vi "Write Qual and SData Masks.vi"(0 "private data":T1={"GTX2_CHANNEL register map"=refnum, "instruction target"=refnum, "channel measure state"=enum."Uninitialized", "in DFE mode?"=FALSE, "prescale"=0, "rx internal data width"=enum."32 Bit", "active point"={"horizontal offset"=0, "vertical offset"=0}, "ut sign"=enum."Positive", "positive counts"={"sample count"=0, "error count"=0}, "negative counts"={"sample count"=0, "error count"=0}}, 11 "error in":errorcluster) -> (4 "private data out":T1={"GTX2_CHANNEL register map"=refnum, "instruction target"=refnum, "channel measure state"=enum."Uninitialized", "in DFE mode?"=FALSE, "prescale"=0, "rx internal data width"=enum."32 Bit", "active point"={"horizontal offset"=0, "vertical offset"=0}, "ut sign"=enum."Positive", "positive counts"={"sample count"=0, "error count"=0}, "negative counts"={"sample count"=0, "error count"=0}}, 15 "error out":errorcluster)   [LabVIEW 2015, in "niHighSpeedSerial Eye Scan Single Point v1 Host.lvclass"]
doc: "Writes the Qualifier and SData masks on the channel.\n\n<B>Input Parameters</B>\n\n<B>private data</B> is the class private data input into the VI.\n\n<B>private data.GTX2_CHANNEL register map</B> is the GTX2 Channel register map to use.\n\n<B>private data.instruction target</B> is the instruction target to use when communicating with the FPGA.\n\n<B>private data.channel measure state</B> maintains the internal state of the Eye Scan Single Point class.\nenum values: Uninitialized,Initialized,Ready,Request,Wait,Read,Process,Finished\n\n<B>private data.in DFE mode?</B> is true if Eye Scan is configured for DFE Equalization Mode.\n\n<B>private data.prescale</B> controls scaling of the sample count in order to keep the sample count and error count within reasonable precision.\n\n<B>private data.receiver data width</B> is the data width (in bits) of the receiver lane.\nenum values: 16 Bit,20 Bit,32 Bit,40 Bit\n\n<B>private data.active point</B> is the point currently being sampled for errors using Eye Scan.\n\n<B>private data.active point.horizontal offset</B> is the horizontal offset of the active point.\n\n<B>private data.active point.vertical offset</B> is the vertical offset of the active point.\n\n<B>private data.ut sign</B> The untapped threshold sign (positive or negative) currently configured on the point being measured.\nPositive is used when in DFE or LPM Equalization Mode, while Negative is only used in DFE Equalization Mode.\n\n<B>private data.positive counts</B> contains the number of sample and error counts measured using the positive UT Sign.\n\n<B>private data.positive counts.sample count</B> is the positive sample count when using DFE mode, or the entire sample count when using LPM mode.\n\n<B>private data.positive counts.error count</B> is the positive error count when using DFE mode, or the entire error count when using LPM mode.\n\n<B>private data.negative counts</B> contains the number of sample and error counts measured using the negative UT Sign.\n\n<B>private data.negative counts.sample count</B> is the negative sample count when using DFE mode, or unused when using LPM mode.\n\n<B>private data.negative counts.error count</B> is the negative error count when using DFE mode, or unused when using LPM mode.\n\n<B>error in</B> describes error conditions that occur before this node runs. This input provides standard 'error in' functionality.\n\n<B>Output Parameters</B>\n\n<B>private data out</B> is the class private data output from the VI.\n\n<B>private data out.GTX2_CHANNEL register map</B> is the register map to use which represents the GTX2 Channel.\n\n<B>private data out.instruction target</B> is the instruction target to use when communicating with the FPGA.\n\n<B>private data out.channel measure state</B> maintains the internal state of the Eye Scan Single Point class.\nenum values: Uninitialized,Initialized,Ready,Request,Wait,Read,Process,Finished\n\n<B>private data out.in DFE mode?</B> is true if Eye Scan is configured for DFE Equalization Mode.\n\n<B>private data out.prescale</B> controls scaling of the sample count in order to keep the sample count and error count within reasonable precision.\n\n<B>private data out.receiver data width</B> is the data width (in bits) of the receiver lane.\nenum values: 16 Bit,20 Bit,32 Bit,40 Bit\n\n<B>private data out.active point</B> is the point currently being sampled for errors using Eye Scan.\n\n<B>private data out.active point.horizontal offset</B> is the horizontal offset of the active point.\n\n<B>private data out.active point.vertical offset</B> is the vertical offset of the active point.\n\n<B>private data out.ut sign</B> contains the number of sample and error counts measured using the positive UT Sign.\nenum values: Positive,Negative\n\n<B>private data out.positive counts</B> contains the number of sample and error counts measured using the positive UT Sign.\n\n<B>private data out.positive counts.sample count</B> is the positive sample count when using DFE mode, or the entire sample count when using LPM mode.\n\n<B>private data out.positive counts.error count</B> is the positive error count when using DFE mode, or the entire error count when using LPM mode.\n\n<B>private data out.negative counts</B> contains the number of sample and error counts measured using the negative UT Sign.\n\n<B>private data out.negative counts.sample count</B> is the negative sample count when using DFE mode, or the entire sample count when using LPM mode.\n\n<B>private data out.negative counts.error count</B> is the negative error count when using DFE mode, or the entire error count when using LPM mode.\n\n<B>error out</B> contains error information. This output provides standard 'error out' functionality."
uses:
  <instrlib>/niHighSpeedSerial/Eye Scan/v1/Host/Impl/Single Point/niHighSpeedSerial Eye Scan Single Point v1 Host.lvclass
  <instrlib>/niHighSpeedSerial/Eye Scan/v1/Host/Impl/Single Point/Private/Private Data.ctl
  <instrlib>/niHighSpeedSerial/Register Maps/Xilinx/v1/Host/GTX2_CHANNEL v1 Host.llb/GTX2_CHANNEL Register Map.lvclass
  <instrlib>/_niInstr/Instruction Framework/v1/Host/Instruction Target/niInstr Instruction Target v1 Host.lvclass
  <instrlib>/niHighSpeedSerial/Eye Scan/v1/Host/Impl/Single Point/Private/Channel Measure State.ctl
  <instrlib>/niHighSpeedSerial/Eye Scan/v1/Host/Common/Public/Data Width.ctl
  <instrlib>/niHighSpeedSerial/Eye Scan/v1/Host/Common/Public/Point Offsets.ctl
  <instrlib>/niHighSpeedSerial/Register Maps/Xilinx/v1/Host/GTX2_CHANNEL v1 Host.llb/ESVertOffsetSign.ctl
  <instrlib>/niHighSpeedSerial/Eye Scan/v1/Host/Impl/Single Point/Private/Counts.ctl
  <instrlib>/niHighSpeedSerial/Register Maps/Xilinx/v1/Host/GTX2_CHANNEL v1 Host.llb/GTX2_CHANNEL Register Map.lvclass/GTX2_CHANNEL Register Map.ctl
  <instrlib>/niHighSpeedSerial/Register Maps/Xilinx/v1/Host/GTX2_CHANNEL v1 Host.llb/Write ES_QUALIFIER_0.vi
  <instrlib>/niHighSpeedSerial/Register Maps/Xilinx/v1/Host/GTX2_CHANNEL v1 Host.llb/Write ES_QUALIFIER_1.vi
  <instrlib>/niHighSpeedSerial/Register Maps/Xilinx/v1/Host/GTX2_CHANNEL v1 Host.llb/Write ES_QUALIFIER_2.vi
  <instrlib>/niHighSpeedSerial/Register Maps/Xilinx/v1/Host/GTX2_CHANNEL v1 Host.llb/Write ES_QUALIFIER_3.vi
  <instrlib>/niHighSpeedSerial/Register Maps/Xilinx/v1/Host/GTX2_CHANNEL v1 Host.llb/Write ES_QUALIFIER_4.vi
  <instrlib>/niHighSpeedSerial/Register Maps/Xilinx/v1/Host/GTX2_CHANNEL v1 Host.llb/Write ES_QUAL_MASK_0.vi
  <instrlib>/niHighSpeedSerial/Register Maps/Xilinx/v1/Host/GTX2_CHANNEL v1 Host.llb/Write ES_QUAL_MASK_1.vi
  <instrlib>/niHighSpeedSerial/Register Maps/Xilinx/v1/Host/GTX2_CHANNEL v1 Host.llb/Write ES_QUAL_MASK_2.vi
  <instrlib>/niHighSpeedSerial/Register Maps/Xilinx/v1/Host/GTX2_CHANNEL v1 Host.llb/Write ES_QUAL_MASK_3.vi
  <instrlib>/niHighSpeedSerial/Register Maps/Xilinx/v1/Host/GTX2_CHANNEL v1 Host.llb/Write ES_QUAL_MASK_4.vi
  <instrlib>/niHighSpeedSerial/Register Maps/Xilinx/v1/Host/GTX2_CHANNEL v1 Host.llb/Write ES_SDATA_MASK_0.vi
  <instrlib>/niHighSpeedSerial/Register Maps/Xilinx/v1/Host/GTX2_CHANNEL v1 Host.llb/Write ES_SDATA_MASK_1.vi
  <instrlib>/niHighSpeedSerial/Register Maps/Xilinx/v1/Host/GTX2_CHANNEL v1 Host.llb/Write ES_SDATA_MASK_2.vi
  <instrlib>/niHighSpeedSerial/Register Maps/Xilinx/v1/Host/GTX2_CHANNEL v1 Host.llb/Write ES_SDATA_MASK_3.vi
  <instrlib>/niHighSpeedSerial/Register Maps/Xilinx/v1/Host/GTX2_CHANNEL v1 Host.llb/Write ES_SDATA_MASK_4.vi
  <instrlib>/niHighSpeedSerial/Register Maps/Xilinx/v1/Host/GTX2_CHANNEL v1 Host.llb/Decode Register to Address.vi
  <instrlib>/_niInstr/Instruction Framework/v1/Host/Instruction Target/Public/Context Write.vi
  <instrlib>/niHighSpeedSerial/Eye Scan/v1/Host/Common/niHighSpeedSerial Eye Scan Common v1 Host.lvlib
  <instrlib>/niHighSpeedSerial/Register Maps/Xilinx/v1/Host/GTX2_CHANNEL v1 Host.llb/GTX2_CHANNEL v1 Host.lvlib
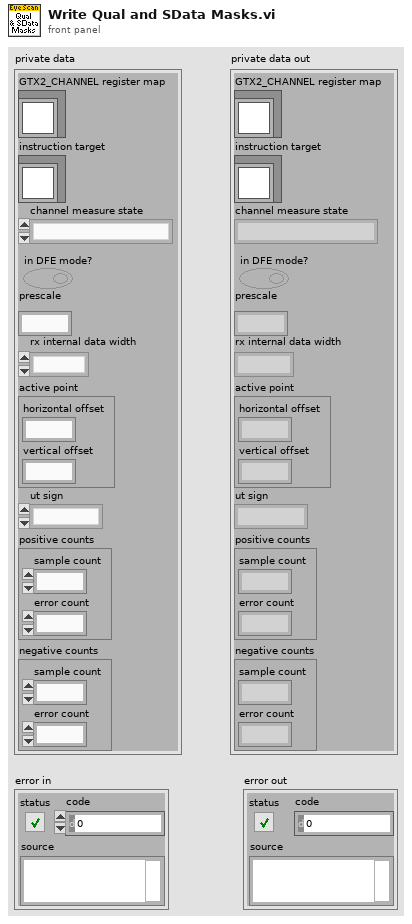
[diagram p1: front panel]
types:
  T1 = typedef "niHighSpeedSerial Eye Scan Single Point v1 Host.lvclass/Private Data.ctl" = cluster{"GTX2_CHANNEL register map":refnum<class "GTX2_CHANNEL Register Map.lvclass">, "instruction target":refnum<class "niInstr Instruction Target v1 Host.lvclass">, "channel measure state":T2, "in DFE mode?":bool, "prescale":u8, "rx internal data width":T3, "active point":T4, "ut sign":T5, "positive counts":T6, "negative counts":T6}
  T2 = typedef "niHighSpeedSerial Eye Scan Single Point v1 Host.lvclass/Channel Measure State.ctl" = enum16{"Uninitialized", "Initialized", "Ready", "Request", "Wait", "Read", "Process", "Finished"}
  T3 = typedef "niHighSpeedSerial Eye Scan Common v1 Host.lvlib/Data Width.ctl" = enum16{"16 Bit", "20 Bit", "32 Bit", "40 Bit"}
  T4 = typedef "niHighSpeedSerial Eye Scan Common v1 Host.lvlib/Point Offsets.ctl" = cluster{"horizontal offset":i16, "vertical offset":i8}
  T5 = typedef "GTX2_CHANNEL v1 Host.lvlib/ESVertOffsetSign.ctl" = enum8{"Positive", "Negative"}
  T6 = typedef "niHighSpeedSerial Eye Scan Single Point v1 Host.lvclass/Counts.ctl" = cluster{"sample count":u64, "error count":u16}
  T7 = cluster{"Qualifier[63:0]":u64, "Qualifier[79:64]":u16, "QualMask[63:0]":u64, "QualMask[79:64]":u16}
  T8 = cluster{"SDataMask[63:0]":u64, "SDataMask[79:64]":u16}
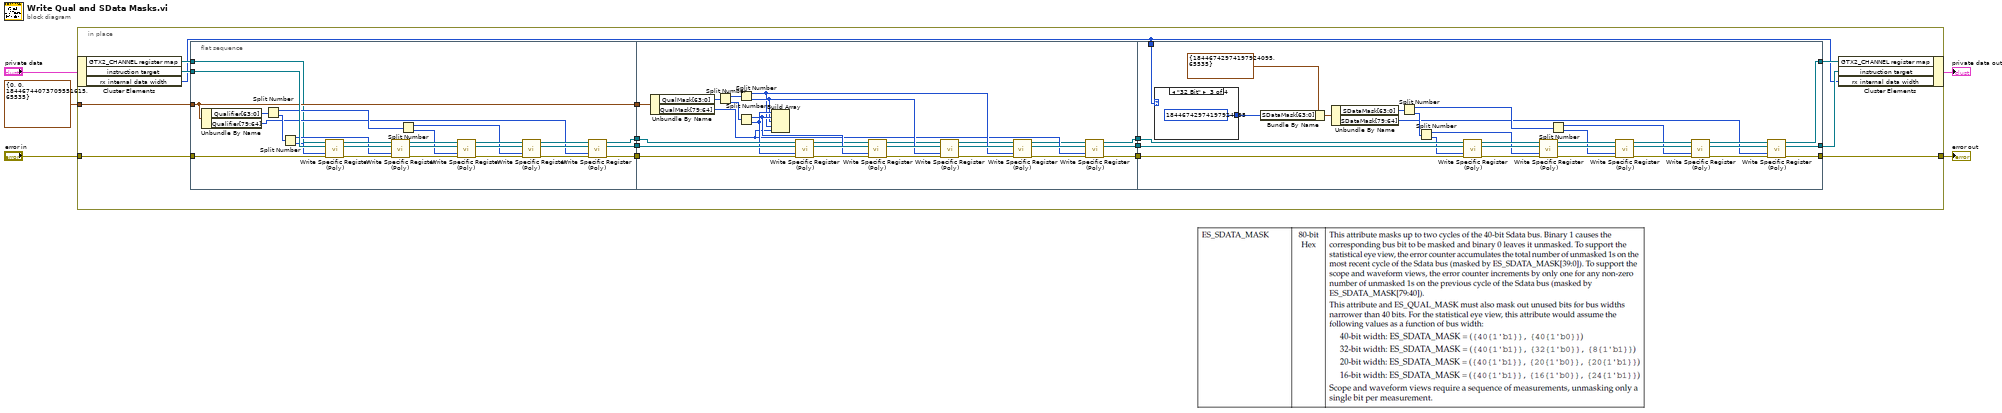
[diagram p0: block diagram]
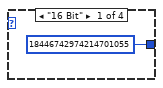
[diagram p2: hidden frame]
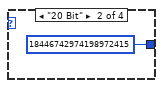
[diagram p3: hidden frame]
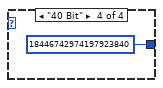
[diagram p4: hidden frame]
diagram:
  n1 = in-place {
    in-place-border: T7 {"Qualifier[63:0]"=0, "Qualifier[79:64]"=0, "QualMask[63:0]"=18446744073709551615, "QualMask[79:64]"=65535} ("Qualifier") -> [w13]
    in-place-border: [w12] -> w1
    in-place-border: "error in" -> [w11]
    n2 = in-place-cluster #1("private data") -> ("GTX2_CHANNEL register map"=w10:refnum<class "GTX2_CHANNEL Register Map.lvclass">, "instruction target"=w9:refnum<class "niInstr Instruction Target v1 Host.lvclass">, "rx internal data width"=w6:T3)
    n3 = flat-sequence {
      tunnel: w9 -> [w47]
      tunnel: w11 -> [w46]
      tunnel: w10 -> [w21]
      tunnel: [w33] -> w20
      tunnel: [w32] -> w19
      tunnel: [w31] -> w18
      tunnel: w13 -> [w22]
      tunnel: [w22] -> w17
      tunnel: w20 -> [w66]
      tunnel: w19 -> [w65]
      tunnel: w18 -> [w61]
      tunnel: [w64] -> w16
      tunnel: [w63] -> w15
      tunnel: [w62] -> w14
      tunnel: w17 -> [w57]
      tunnel: w16 -> [w104]
      tunnel: w15 -> [w103]
      tunnel: w14 -> [w102]
      tunnel: [w89] -> w12
      tunnel: [w80] -> w7
      tunnel: [w79] -> w8
      tunnel: w6 -> [w76]
      frame #0 {
        n4 = Unbundle By Name(w22) -> ("Qualifier[63:0]"=w28:u64, "Qualifier[79:64]"=w23:u16)
        n5 = Split Number(x=w28) -> (hi(x)=w29:u32, lo(x)=w30:u32)
        n6 = Split Number(x=w30) -> (hi(x)=w26:u16, lo(x)=w27:u16)
        n7 = call-poly <instrlib>:"Write Specific Register (Poly).vi"("gtx2_channel register map object in"=w21, "instruction target in"=w47, "ES_QUALIFIER_0"=w27, "error in"=w46) -> ("gtx2_channel register map object out"=w45:refnum<class "GTX2_CHANNEL Register Map.lvclass">, "instruction target out"=w44:refnum<class "niInstr Instruction Target v1 Host.lvclass">, "error out"=w43:errorcluster)  [unwired: 9 in]
        n8 = call-poly <instrlib>:"Write Specific Register (Poly).vi"("gtx2_channel register map object in"=w45, "instruction target in"=w44, "ES_QUALIFIER_1"=w26, "error in"=w43) -> ("gtx2_channel register map object out"=w42:refnum<class "GTX2_CHANNEL Register Map.lvclass">, "instruction target out"=w41:refnum<class "niInstr Instruction Target v1 Host.lvclass">, "error out"=w40:errorcluster)  [unwired: 9 in]
        n9 = Split Number(x=w29) -> (hi(x)=w24:u16, lo(x)=w25:u16)
        n10 = call-poly <instrlib>:"Write Specific Register (Poly).vi"("gtx2_channel register map object in"=w42, "instruction target in"=w41, "ES_QUALIFIER_2"=w25, "error in"=w40) -> ("gtx2_channel register map object out"=w38:refnum<class "GTX2_CHANNEL Register Map.lvclass">, "instruction target out"=w37:refnum<class "niInstr Instruction Target v1 Host.lvclass">, "error out"=w39:errorcluster)  [unwired: 9 in]
        n11 = call-poly <instrlib>:"Write Specific Register (Poly).vi"("gtx2_channel register map object in"=w38, "instruction target in"=w37, "ES_QUALIFIER_3"=w24, "error in"=w39) -> ("gtx2_channel register map object out"=w36:refnum<class "GTX2_CHANNEL Register Map.lvclass">, "instruction target out"=w35:refnum<class "niInstr Instruction Target v1 Host.lvclass">, "error out"=w34:errorcluster)  [unwired: 9 in]
        n12 = call-poly <instrlib>:"Write Specific Register (Poly).vi"("gtx2_channel register map object in"=w36, "instruction target in"=w35, "ES_QUALIFIER_4"=w23, "error in"=w34) -> ("gtx2_channel register map object out"=w33:refnum<class "GTX2_CHANNEL Register Map.lvclass">, "instruction target out"=w32:refnum<class "niInstr Instruction Target v1 Host.lvclass">, "error out"=w31:errorcluster)  [unwired: 9 in]
      }
      frame #1 {
        n13 = Unbundle By Name(w57) -> ("QualMask[63:0]"=w60:u64, "QualMask[79:64]"=w52:u16)
        n14 = Split Number(x=w60) -> (hi(x)=w58:u32, lo(x)=w59:u32)
        n15 = Split Number(x=w58) -> (hi(x)=w53:u16, lo(x)=w54:u16)
        n16 = Split Number(x=w59) -> (hi(x)=w55:u16, lo(x)=w56:u16)
        n17 = Build Array(w56, w55, w54, w53, w52) -> ()  [unwired: 1 out]
        n18 = call-poly <instrlib>:"Write Specific Register (Poly).vi"("gtx2_channel register map object in"=w66, "instruction target in"=w65, "ES_QUAL_MASK_0"=w56, "error in"=w61) -> ("gtx2_channel register map object out"=w48:refnum<class "GTX2_CHANNEL Register Map.lvclass">, "instruction target out"=w67:refnum<class "niInstr Instruction Target v1 Host.lvclass">, "error out"=w68:errorcluster)  [unwired: 9 in]
        n19 = call-poly <instrlib>:"Write Specific Register (Poly).vi"("gtx2_channel register map object in"=w48, "instruction target in"=w67, "ES_QUAL_MASK_1"=w55, "error in"=w68) -> ("gtx2_channel register map object out"=w49:refnum<class "GTX2_CHANNEL Register Map.lvclass">, "instruction target out"=w69:refnum<class "niInstr Instruction Target v1 Host.lvclass">, "error out"=w70:errorcluster)  [unwired: 9 in]
        n20 = call-poly <instrlib>:"Write Specific Register (Poly).vi"("gtx2_channel register map object in"=w49, "instruction target in"=w69, "ES_QUAL_MASK_2"=w54, "error in"=w70) -> ("gtx2_channel register map object out"=w50:refnum<class "GTX2_CHANNEL Register Map.lvclass">, "instruction target out"=w73:refnum<class "niInstr Instruction Target v1 Host.lvclass">, "error out"=w74:errorcluster)  [unwired: 9 in]
        n21 = call-poly <instrlib>:"Write Specific Register (Poly).vi"("gtx2_channel register map object in"=w50, "instruction target in"=w73, "ES_QUAL_MASK_3"=w53, "error in"=w74) -> ("gtx2_channel register map object out"=w51:refnum<class "GTX2_CHANNEL Register Map.lvclass">, "instruction target out"=w72:refnum<class "niInstr Instruction Target v1 Host.lvclass">, "error out"=w71:errorcluster)  [unwired: 9 in]
        n22 = call-poly <instrlib>:"Write Specific Register (Poly).vi"("gtx2_channel register map object in"=w51, "instruction target in"=w72, "ES_QUAL_MASK_4"=w52, "error in"=w71) -> ("gtx2_channel register map object out"=w64:refnum<class "GTX2_CHANNEL Register Map.lvclass">, "instruction target out"=w63:refnum<class "niInstr Instruction Target v1 Host.lvclass">, "error out"=w62:errorcluster)  [unwired: 9 in]
      }
      frame #2 {
        n23 = case shown="\"32 Bit\"" w76 {
          tunnel: [u64 18446742974214701055 ("SDataMask[63:0]") u64 18446742974198972415 ("SDataMask[63:0]") u64 18446742974197924095 ("SDataMask[63:0]") u64 18446742974197923840 ("SDataMask[63:0]")] -> w75
          frame "16 Bit" {
          }
          frame "20 Bit" {
          }
          frame "32 Bit" {
          }
          frame "40 Bit" {
          }
        }
        n24 = Bundle By Name(cluster=T8 {"SDataMask[63:0]"=18446742974197924095, "SDataMask[79:64]"=65535} ("SDataMask"), "SDataMask[63:0]"=w75) -> (w77:T8)
        n25 = Unbundle By Name(w77) -> ("SDataMask[63:0]"=w86:u64, "SDataMask[79:64]"=w81:u16)
        n26 = Split Number(x=w86) -> (hi(x)=w87:u32, lo(x)=w88:u32)
        n27 = Split Number(x=w88) -> (hi(x)=w84:u16, lo(x)=w85:u16)
        n28 = call-poly <instrlib>:"Write Specific Register (Poly).vi"("gtx2_channel register map object in"=w104, "instruction target in"=w103, "ES_SDATA_MASK_0"=w85, "error in"=w102) -> ("gtx2_channel register map object out"=w100:refnum<class "GTX2_CHANNEL Register Map.lvclass">, "instruction target out"=w99:refnum<class "niInstr Instruction Target v1 Host.lvclass">, "error out"=w101:errorcluster)  [unwired: 9 in]
        n29 = call-poly <instrlib>:"Write Specific Register (Poly).vi"("gtx2_channel register map object in"=w100, "instruction target in"=w99, "ES_SDATA_MASK_1"=w84, "error in"=w101) -> ("gtx2_channel register map object out"=w97:refnum<class "GTX2_CHANNEL Register Map.lvclass">, "instruction target out"=w96:refnum<class "niInstr Instruction Target v1 Host.lvclass">, "error out"=w98:errorcluster)  [unwired: 9 in]
        n30 = Split Number(x=w87) -> (hi(x)=w82:u16, lo(x)=w83:u16)
        n31 = call-poly <instrlib>:"Write Specific Register (Poly).vi"("gtx2_channel register map object in"=w97, "instruction target in"=w96, "ES_SDATA_MASK_2"=w83, "error in"=w98) -> ("gtx2_channel register map object out"=w95:refnum<class "GTX2_CHANNEL Register Map.lvclass">, "instruction target out"=w94:refnum<class "niInstr Instruction Target v1 Host.lvclass">, "error out"=w93:errorcluster)  [unwired: 9 in]
        n32 = call-poly <instrlib>:"Write Specific Register (Poly).vi"("gtx2_channel register map object in"=w95, "instruction target in"=w94, "ES_SDATA_MASK_3"=w82, "error in"=w93) -> ("gtx2_channel register map object out"=w92:refnum<class "GTX2_CHANNEL Register Map.lvclass">, "instruction target out"=w91:refnum<class "niInstr Instruction Target v1 Host.lvclass">, "error out"=w90:errorcluster)  [unwired: 9 in]
        n33 = call-poly <instrlib>:"Write Specific Register (Poly).vi"("gtx2_channel register map object in"=w92, "instruction target in"=w91, "ES_SDATA_MASK_4"=w81, "error in"=w90) -> ("gtx2_channel register map object out"=w79:refnum<class "GTX2_CHANNEL Register Map.lvclass">, "instruction target out"=w80:refnum<class "niInstr Instruction Target v1 Host.lvclass">, "error out"=w89:errorcluster)  [unwired: 9 in]
      }
    }
    n34 = in-place-cluster #1("GTX2_CHANNEL register map"=w8, "instruction target"=w7, "rx internal data width"=w6) -> (→"private data out":T1)
  }
  "error out" <- w1
